vi "Factory Core.vi"(8 "error in (no error)":errorcluster, 11 "File Parser Interface in":refnum<class "File Parser Interface.lvclass">) -> (0 "error out":errorcluster, 3 "File Parser Interface out":refnum<class "File Parser Interface.lvclass">)   [LabVIEW 2018, in "File Parser Interface.lvlib" / "File Parser Interface.lvclass"]
uses:
  File Parser Interface.lvclass
  FPF.lvlibp/Factory Plugin Framework.lvclass
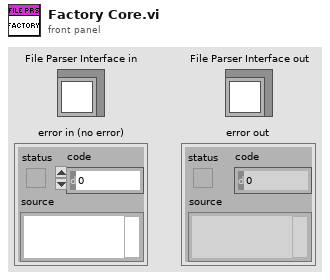
[diagram p1: front panel]
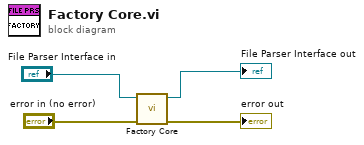
[diagram p0: block diagram]
diagram:
  n1 = call-parent "Factory Core.vi"("error in (no error)"="error in (no error)", "Factory Plugin Framework in"="File Parser Interface in") -> ("error out"=→"error out":errorcluster, "Factory Plugin Framework out"=→"File Parser Interface out":refnum<class "File Parser Interface.lvclass">)  [unwired: 8 in]
